vi "Initial Condition (DBL Array).vi"(2 "initialize":bool, 3 "Initial Conditions":dbl[](array[numeric]) format="%.2f", 5 "Input Points":dbl[](array[numeric]) format="%.2f") -> (1 "Output Points":dbl[](array[numeric]) format="%.2f")   [LabVIEW 2020, in "NI_AdvCtrl_nonlinear.lvlib"]
doc: "LabVIEW no longer supports this VI. You can obtain similar functionality by installing the LabVIEW Simulation Module.\n\nProduces a predefined initial condition only during the first iteration of the control or simulation task."
uses:
  <vilib>/addons/control/advanced/NI_AdvCtrl_nonlinear.lvlib
  <vilib>/addons/control/advanced/NI_AdvCtrl_continuous linear.lvlib
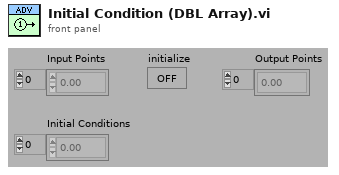
[diagram p1: front panel]
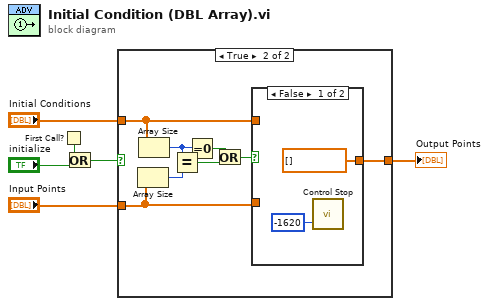
[diagram p0: block diagram]
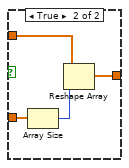
[diagram p3: hidden frame]
diagram:
  n1 = First Call?() -> (First Call?: T/F=w6:bool)
  n2 = Or(x=w6, y="initialize") -> (x .or. y?=w4:bool)
  n3 = case shown="True" w4 {
    tunnel: "Input Points" -> [w7 w11]
    tunnel: [w7 w15] -> w2
    tunnel: "Initial Conditions" -> [_ w12]
    frame False {
    }
    frame True {
      n4 = Array Size(array=w11) -> (size(s)=w14:i32)
      n5 = Array Size(array=w12) -> (size(s)=w8:i32)
      n6 = Equal?(x=w8, y=w14) -> (x = y?=w13:bool)
      n7 = Equal To 0?(x=w8) -> (x = 0?=w9:bool)
      n8 = Or(x=w9, y=w13) -> (x .or. y?=w10:bool)
      n9 = case shown="False" w10 {
        tunnel: w11 -> [_ w21]
        tunnel: w12 -> [_ w19]
        tunnel: [dbl[] [] ("Initial Conditions") w18] -> w15
        frame False {
          n10 = call <vilib>:"Control Stop.vi"("error"=-1620) -> ()  [unwired: 2 out]
        }
        frame True {
          n11 = Array Size(array=w21) -> (size(s)=w20:i32)
          n12 = Reshape Array(w19, w20) -> (w18:dbl[])
        }
      }
    }
  }
  "Output Points" <- w2
